vi "evaluate_gear_data_read.vi"(4 "active_batch_code":string, 6 "current_access_level":i32, 8 "current_batch_ID":string, 9 "NOK_stations":string[](array[string]), 10 "part_number_ref_status":string, 11 "enqueued_states_in":T1[](array[typedef])) -> (3 "enqueued_states_out":T1[](array[typedef]))   [LabVIEW 2019]
uses:
  queues/typedef/DOCK_MAIN_queue_element.ctl
  DOCK_MAIN_sequence_state.ctl
  FGV/controls_state/FGV_DOCK_controls_state.ctl
  FGV/DOCK_multistate_indicator/FGV_DOCK_multistate_indicator.ctl
  FGV/DOCK_records_display/FGV_DOCK_records_display.ctl
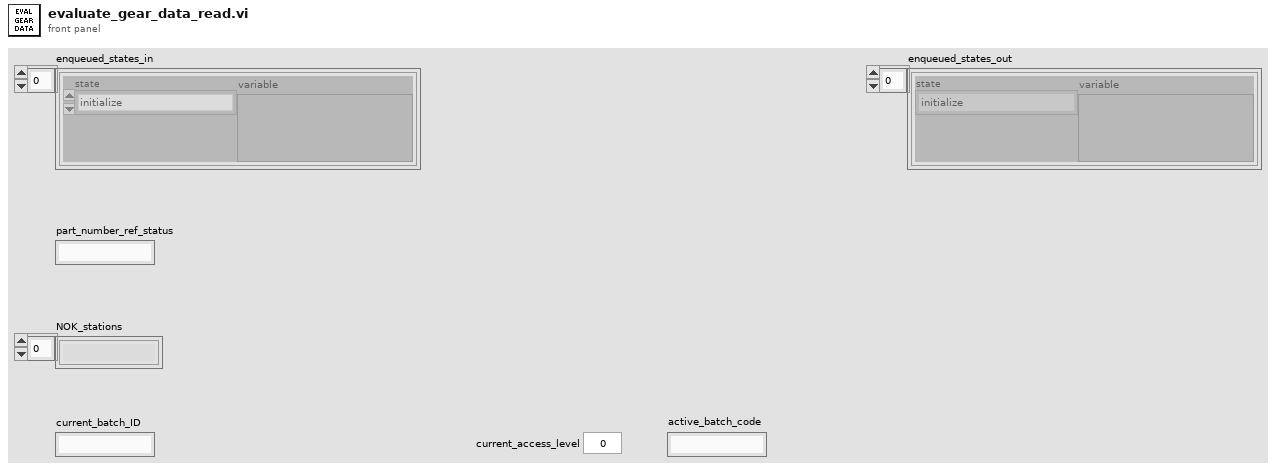
[diagram p1: front panel]
types:
  T1 = typedef "DOCK_MAIN_queue_element.ctl" = cluster{"state":T2, "variable":variant}
  T2 = typedef "DOCK_MAIN_sequence_state.ctl" = enum16{"initialize", "get_next_state", "USER_login", "USER_logout", "read_reference_list", "read_batch_size_list", "change_reference", "start_batch", "reload_batch", "finish_batch?", "finish_batch", "preread_gear_data_check", "read_gear_data", "refresh_gear_data", "save_gear_to_batch", "clear_gear_data", "print_label", "report_get", "error", "stop"}
  T3 = typedef "FGV_DOCK_multistate_indicator.ctl" = enum16{"initialize", "login", "logout", "start_batch", "finish_batch", "gear_OK", "gear_NOK", "gear_clear", "translate", "error", "error_clear"}
  T4 = typedef "FGV_DOCK_controls_state.ctl" = enum16{"initialize", "login_event", "translation_event", "batch_event", "reload_event", "gear_event", "gear_saved_event", "gear_in_another_batch_event", "gear_in_current_batch_event", "NOK_ref_gear_event", "NOK_station_gear_event", "get_gear_loaded_status"}
  T5 = typedef "FGV_DOCK_records_display.ctl" = enum16{"initialize", "set_reference_data", "set_serial", "set_header", "set_operations", "set_results", "set_batches", "get_reference_data", "get_part_number_ref", "get_serial", "get_batch_code", "get_gear_ID", "get_operation_IDs", "toggle_results", "show_all_results", "hide_all_results", "display", "clear"}
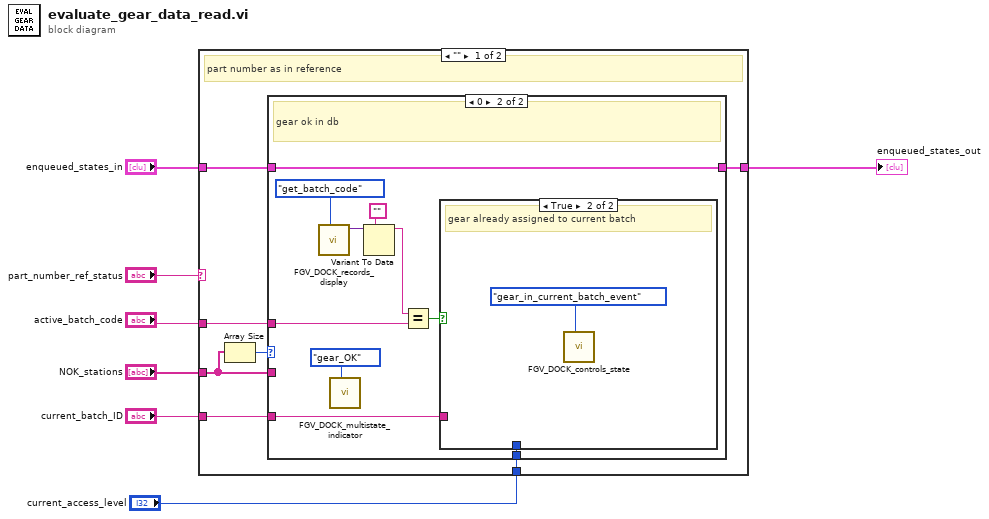
[diagram p0: block diagram]
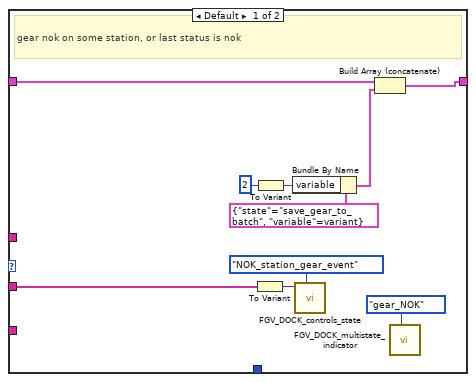
[diagram p2: hidden frame]
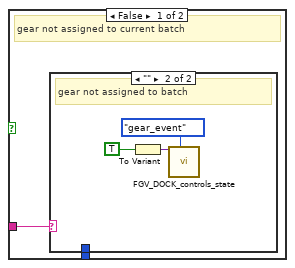
[diagram p3: hidden frame]
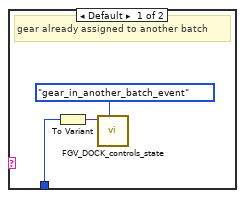
[diagram p4: hidden frame]
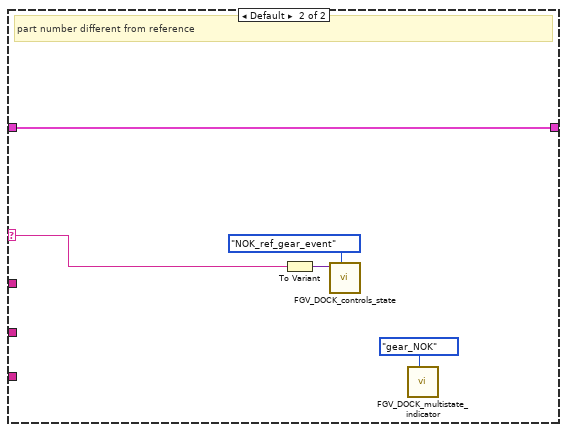
[diagram p5: hidden frame]
diagram:
  n1 = case shown="\"\"" "part_number_ref_status" {
    selector: "part_number_ref_status" -> [_ w46]
    tunnel: "NOK_stations" -> [w13 _]
    tunnel: "enqueued_states_in" -> [w12 w45]
    tunnel: [w11 w45] -> w7
    tunnel: "current_batch_ID" -> [w10 _]
    tunnel: "current_access_level" -> [w9 _]
    tunnel: "active_batch_code" -> [w8 _]
    frame "" {
      # "part number as in reference"
      n2 = Array Size(array=w13) -> (size(s)=w14:i32)
      n3 = case shown="0" w14 {
        tunnel: w13 -> [w22 _]
        tunnel: w12 -> [w21 w34]
        tunnel: [w20 w34] -> w11
        tunnel: w10 -> [_ w33]
        tunnel: w9 -> [_ w32]
        tunnel: w8 -> [_ w25]
        frame Default {
          # "gear nok on some station, or last status is nok"
          n4 = To Variant(anything=w22) -> (Variant=w23:variant)
          n5 = To Variant(anything=2) -> (Variant=w19:variant)
          n6 = Bundle By Name(cluster=T1 {"state"=enum."save_gear_to_batch", "variable"=variant} ("element"), "variable"=w19) -> (w16:T1)
          n7 = call "FGV_DOCK_controls_state.vi"("options"=FGV_DOCK_controls_state."NOK_station_gear_event", "input"=w23) -> ()  [unwired: 8 in, 2 out]
          n8 = Build Array (concatenate)(w21, w16) -> (w20:T1[])
          n9 = call "FGV_DOCK_multistate_indicator.vi"("options"=FGV_DOCK_multistate_indicator."gear_NOK") -> ()  [unwired: 10 in, 1 out]
        }
        frame 0 {
          # "gear ok in db"
          n10 = call "FGV_DOCK_records_display.vi"("options"=FGV_DOCK_records_display."get_batch_code") -> ("output"=w29:variant)  [unwired: 9 in, 1 out]
          n11 = call "FGV_DOCK_multistate_indicator.vi"("options"=FGV_DOCK_multistate_indicator."gear_OK") -> ()  [unwired: 10 in, 1 out]
          n12 = Variant To Data(type="", Variant=w29) -> (data=w26:string)  [unwired: 1 in, 1 out]
          n13 = Equal?(x=w26, y=w25) -> (x = y?=w27:bool)
          n14 = case shown="True" w27 {
            tunnel: w33 -> [w36 _]
            tunnel: w32 -> [w35 _]
            frame False {
              # "gear not assigned to current batch"
              n15 = case shown="\"\"" w36 {
                tunnel: w35 -> [w37 _]
                frame Default {
                  # "gear already assigned to another batch"
                  n16 = To Variant(anything=w37) -> (Variant=w38:variant)
                  n17 = call "FGV_DOCK_controls_state.vi"("options"=FGV_DOCK_controls_state."gear_in_another_batch_event", "input"=w38) -> ()  [unwired: 8 in, 2 out]
                }
                frame "" {
                  # "gear not assigned to batch"
                  n18 = To Variant(anything=TRUE) -> (Variant=w41:variant)
                  n19 = call "FGV_DOCK_controls_state.vi"("options"=FGV_DOCK_controls_state."gear_event", "input"=w41) -> ()  [unwired: 8 in, 2 out]
                }
              }
            }
            frame True {
              # "gear already assigned to current batch"
              n20 = call "FGV_DOCK_controls_state.vi"("options"=FGV_DOCK_controls_state."gear_in_current_batch_event") -> ()  [unwired: 9 in, 2 out]
            }
          }
        }
      }
    }
    frame Default {
      # "part number different from reference"
      n21 = To Variant(anything=w46) -> (Variant=w47:variant)
      n22 = call "FGV_DOCK_controls_state.vi"("options"=FGV_DOCK_controls_state."NOK_ref_gear_event", "input"=w47) -> ()  [unwired: 8 in, 2 out]
      n23 = call "FGV_DOCK_multistate_indicator.vi"("options"=FGV_DOCK_multistate_indicator."gear_NOK") -> ()  [unwired: 10 in, 1 out]
    }
  }
  "enqueued_states_out" <- w7
